vi "My VI.vi"() -> ()   [LabVIEW 2015]
panel:
  out "number (0 to 1)":dbl
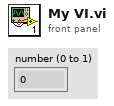
[diagram p1: front panel]
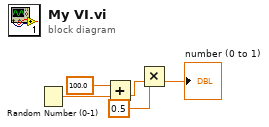
[diagram p0: block diagram]
diagram:
  n1 = Random Number (0-1)() -> (number: 0 to 1=w5:dbl)
  n2 = Add(x=100.0, y=w5) -> (x+y=w4:dbl)
  n3 = Multiply(x=0.5, y=w4) -> (x*y=→"number (0 to 1)":dbl)
